vi "Read Sum.vi"(11 "Self Incrementer in":refnum<class "Self Incrementer.lvclass">) -> (2 "Sum":dbl, 3 "Self Incrementer in":refnum<class "Self Incrementer.lvclass">)   [LabVIEW 2020, in "Messaging Tests.lvlib" / "Self Incrementer.lvclass"]
uses:
  Self Incrementer.lvclass
  Self Incrementer.lvclass/Self Incrementer.ctl
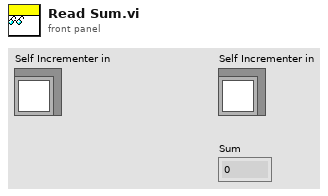
[diagram p1: front panel]
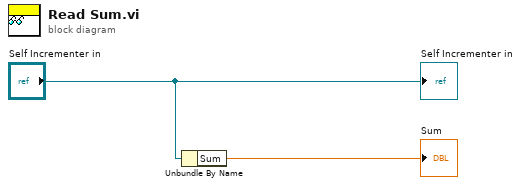
[diagram p0: block diagram]
diagram:
  n1 = Unbundle By Name("Self Incrementer in") -> ("Sum"=→"Sum":dbl)
  "Self Incrementer in" <- "Self Incrementer in"
